vi "ServiceModeTest2.vi"(7 "Erd_KeyPersonality ERD #":T1={"ERD Number"=63232, "Data Type"=enum."string"} {"ERD Number" format="%.0x"}, 8 "Error In":errorcluster, 9 "UI GEA Inputs":T3={"Source"=228, "Destination"=37} {"Destination" format="%.0x"; "Source" format="%.0x"}, 10 "MC GEA Inputs":T3={"Source"=228, "Destination"=36} {"Destination" format="%.0x"; "Source" format="%.0x"}, 11 "GEA2 Reference In":refnum<k24>) -> (0 "Error Out":errorcluster, 1 "Report Text":string, 2 "Pass/Fail?":bool, 3 "GEA2 Reference Out":refnum<k24>)   [LabVIEW 2016]
uses:
  Q:/Common/DLLs/GEA3/GeaCommunication.dll
  Common/DLLs/GEA3/GeaCommunication.dll
  Common/LabVIEW GEA2 Toolkit/LabVIEW_GEA2_Toolkit.lvlibp/type defs/Source_Destination.ctl
  Common/LabVIEW GEA2 Toolkit/LabVIEW_GEA2_Toolkit.lvlibp/type defs/ERD Read Data In.ctl
  Common/LabVIEW GEA2 Toolkit/LabVIEW_GEA2_Toolkit.lvlibp/type defs/Data Type.ctl
  Centauro Washer/Product Testcode/Centauro/Valew Common/type defs/LED Status OOB.ctl
  Common/Type Defs/JL_Buttons.ctl
  Common/LabVIEW GEA2 Toolkit/LabVIEW_GEA2_Toolkit.lvlibp
panel:
  in  "Board Index":i32
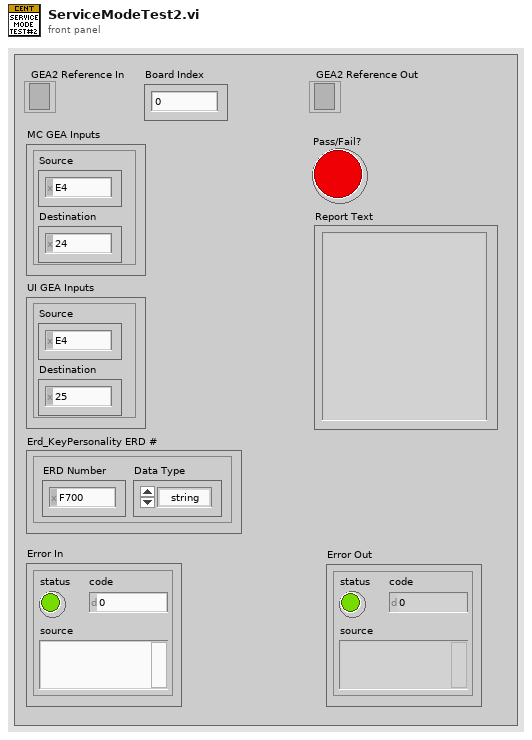
[diagram p1: front panel]
types:
  T1 = typedef "LabVIEW_GEA2_Toolkit.lvlibp/ERD Read Data In.ctl" = cluster{"ERD Number":u16, "Data Type":T2}
  T2 = typedef "LabVIEW_GEA2_Toolkit.lvlibp/Data Type.ctl" = enum16{"string", "boolean", "uint8_t", "uint16_t", "uint32_t", "uint64_t", "int8_t", "int16_t", "int32_t", "int64_t"}
  T3 = typedef "LabVIEW_GEA2_Toolkit.lvlibp/Source_Destination.ctl" = cluster{"Source":u8, "Destination":u8}
  T4 = typedef "JL_Buttons.ctl" = enum16{"Power", "Start / Pause ", "Temp Option ", "Dryness Level", "Time Option", "Time Increment ", "Time Decrement ", "MyCycle", "eDry ", "Delay", "Extended Tumble", "Control Lock", "Volume/Signal", "Damp Alert / Drum Light", "Unused", "(SW213)", "(SW322)", "Clear / Reset"}
  T5 = typedef "LED Status OOB.ctl" = enum32{"Off", "On", "Blink"}
  T6 = cluster{"Damp":T5, "Dry":T5, "Cool":T5, "Eco":T5}
  T7 = typedef "LabVIEW_GEA2_Toolkit.lvlibp/ERD Read Data Out.ctl" = cluster{"ERD Number":u16, "Data":string}
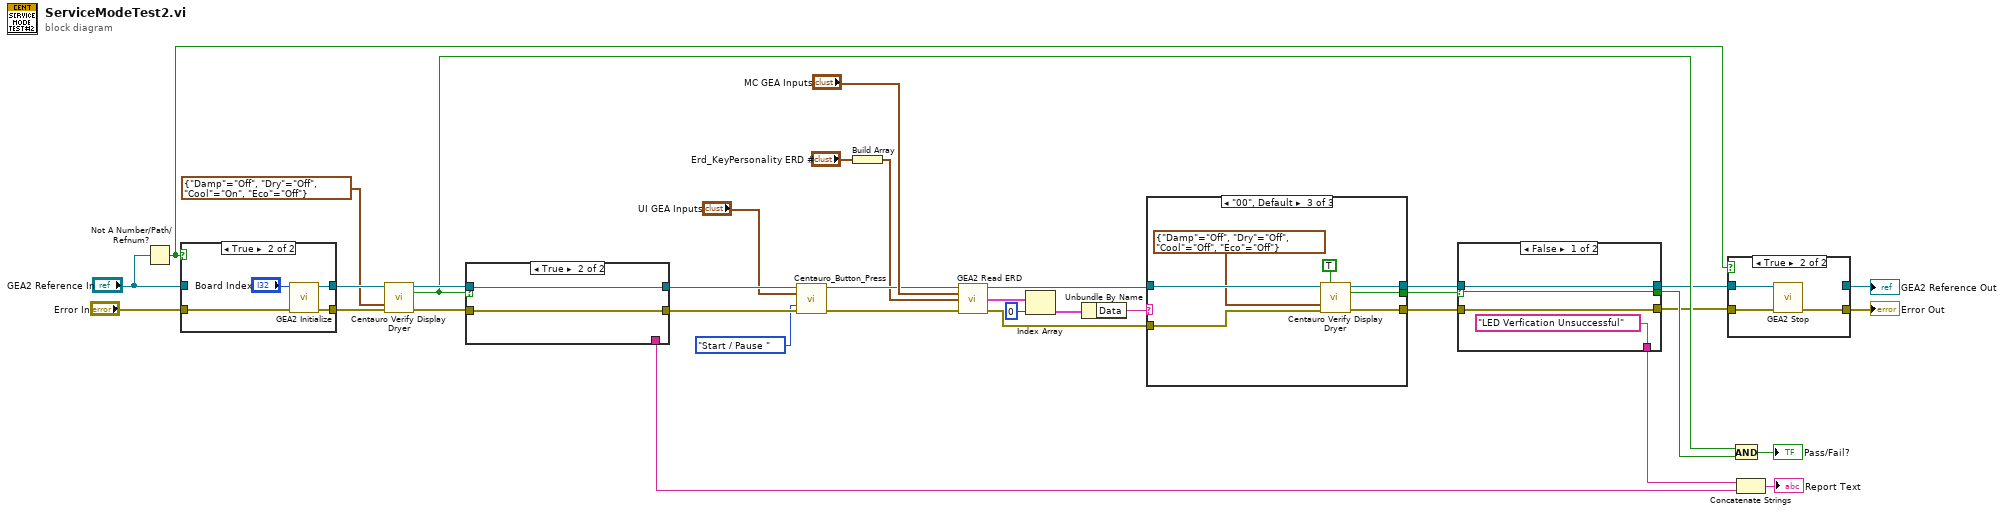
[diagram p0: block diagram]
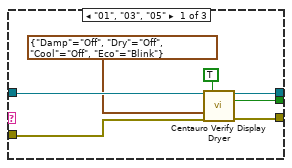
[diagram p4: hidden frame]
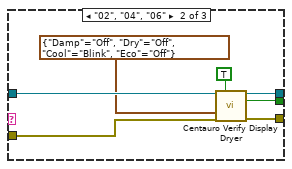
[diagram p5: hidden frame]
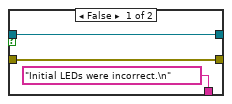
[diagram p6: hidden frame]
diagram:
  n1 = Not A Number/Path/Refnum?(number/path/refnum="GEA2 Reference In") -> (NaN/Path/Refnum?=w4:bool)
  n2 = case shown="True" w4 {
    tunnel: [w37 w42] -> w33
    tunnel: "Error In" -> [w37 w41]
    tunnel: [w38 w40] -> w34
    tunnel: "GEA2 Reference In" -> [w38 _]
    frame False {
    }
    frame True {
      n3 = call "GEA2 Initialize.vi"("Board Index"="Board Index", "error in"=w41) -> ("GEA2 Reference Out"=w40:refnum<k24>, "error out"=w42:errorcluster)  [unwired: 11 in, 1 out]
    }
  }
  n4 = call "Centauro Verify Display Dryer.vi"("GEA2 Reference In"=w34, "Expected LED Status"=T6 {"Damp"=enum."Off", "Dry"=enum."Off", "Cool"=enum."On", "Eco"=enum."Off"}, "Error In"=w33) -> ("GEA2 Reference Out"=w32:refnum<k24>, "Pass/Fail?"=w23:bool, "Error Out"=w31:errorcluster)  [unwired: 7 in, 3 out]
  n5 = case shown="True" w23 {
    tunnel: w32 -> [w45 w47]
    tunnel: [w45 w47] -> w16
    tunnel: [w44 w46] -> w15
    tunnel: w31 -> [w44 w46]
    tunnel: ["Initial LEDs were incorrect.\n" _] -> w18
    frame False {
    }
    frame True {
    }
  }
  n6 = call "Centauro_Button_Press.vi"("GEA2 Reference In"=w16, "GEA Inputs"="UI GEA Inputs", "Button"=JL_Buttons."Start / Pause ", "Error In"=w15) -> ("GEA2 Reference Out"=w14:refnum<k24>, "Error Out"=w13:errorcluster)  [unwired: 10 in]
  n7 = Build Array("Erd_KeyPersonality ERD #") -> (w2:T1[])
  n8 = call "GEA2 Read ERD.vi"("GEA2 Reference In"=w14, "GEA Inputs"="MC GEA Inputs", "Read ERD List"=w2, "Error In"=w13) -> ("GEA2 Reference Out"=w25:refnum<k24>, "ERD Data Out"=w29:T7[], "Error Out"=w24:errorcluster)  [unwired: 8 in, 1 out]
  n9 = Index Array(array=w29, index=0) -> (element=w27:T7)
  n10 = Unbundle By Name(w27) -> ("Data"=w26:string)
  n11 = case shown="\"00\", Default" w26 {
    tunnel: w25 -> [w53 w61 w68]
    tunnel: w24 -> [w54 w60 w67]
    tunnel: [w52 w59 w66] -> w22
    tunnel: [w51 w58 w65] -> w8
    tunnel: [w50 w57 w64] -> w6
    frame "01", "03", "05" {
      n12 = call "Centauro Verify Display Dryer.vi"("GEA2 Reference In"=w53, "Service Mode?"=TRUE, "Expected LED Status"=T6 {"Damp"=enum."Off", "Dry"=enum."Off", "Cool"=enum."Off", "Eco"=enum."Blink"}, "Error In"=w54) -> ("GEA2 Reference Out"=w51:refnum<k24>, "Pass/Fail?"=w52:bool, "Error Out"=w50:errorcluster)  [unwired: 6 in, 3 out]
    }
    frame "02", "04", "06" {
      n13 = call "Centauro Verify Display Dryer.vi"("GEA2 Reference In"=w61, "Service Mode?"=TRUE, "Expected LED Status"=T6 {"Damp"=enum."Off", "Dry"=enum."Off", "Cool"=enum."Blink", "Eco"=enum."Off"}, "Error In"=w60) -> ("GEA2 Reference Out"=w58:refnum<k24>, "Pass/Fail?"=w59:bool, "Error Out"=w57:errorcluster)  [unwired: 6 in, 3 out]
    }
    frame "00", Default {
      n14 = call "Centauro Verify Display Dryer.vi"("GEA2 Reference In"=w68, "Service Mode?"=TRUE, "Expected LED Status"=T6 {"Damp"=enum."Off", "Dry"=enum."Off", "Cool"=enum."Off", "Eco"=enum."Off"}, "Error In"=w67) -> ("GEA2 Reference Out"=w65:refnum<k24>, "Pass/Fail?"=w66:bool, "Error Out"=w64:errorcluster)  [unwired: 6 in, 3 out]
    }
  }
  n15 = case shown="False" w22 {
    selector: w22 -> [w71 w75]
    tunnel: [w71 w75] -> w21
    tunnel: ["LED Verfication Unsuccessful" _] -> w19
    tunnel: w8 -> [w70 w74]
    tunnel: [w70 w74] -> w7
    tunnel: [w69 w73] -> w5
    tunnel: w6 -> [w69 w73]
    frame False {
    }
    frame True {
    }
  }
  n16 = case shown="True" w4 {
    tunnel: [w76 w80] -> w10
    tunnel: w7 -> [w77 w79]
    tunnel: w5 -> [w76 w78]
    tunnel: [w77 _] -> w9
    frame False {
    }
    frame True {
      n17 = call "GEA2 Stop.vi"("GEA2 Reference In"=w79, "Error In"=w78) -> ("Error Out"=w80:errorcluster)  [unwired: 13 in]
    }
  }
  "GEA2 Reference Out" <- w9
  "Error Out" <- w10
  n18 = And(x=w23, y=w21) -> (x .and. y?=→"Pass/Fail?":bool)
  n19 = Concatenate Strings(w19, w18) -> (→"Report Text":string)
